vi "PathPlanningSim.vi"() -> ()   [LabVIEW 2019]
uses:
  <vilib>/Analysis/6fits.llb/nD B-Spline Fit.vi
  <vilib>/robotics/Navigation/shared/WorldMap/OccupancyGridWorldMap/NI_Robotics_OccupancyGridWorldMap.lvclass
  <vilib>/Analysis/NI_AALPro.lvlib
panel:
  out "Array":dbl[](array[numeric])
  out "A* Planned\nPath Coordinates":dbl[][](array[numeric])
  in  "stop":bool
  out "Real Occupancy Grid":dbl[][](array[numeric])
  out "Trajectory Plot":cluster{dbl[], dbl[]}[](graph)
  out "Intensity Graph 2":dbl[][](graph) caption="Intensity Graph"
  # "x coordinates"
  # "y coordinates"
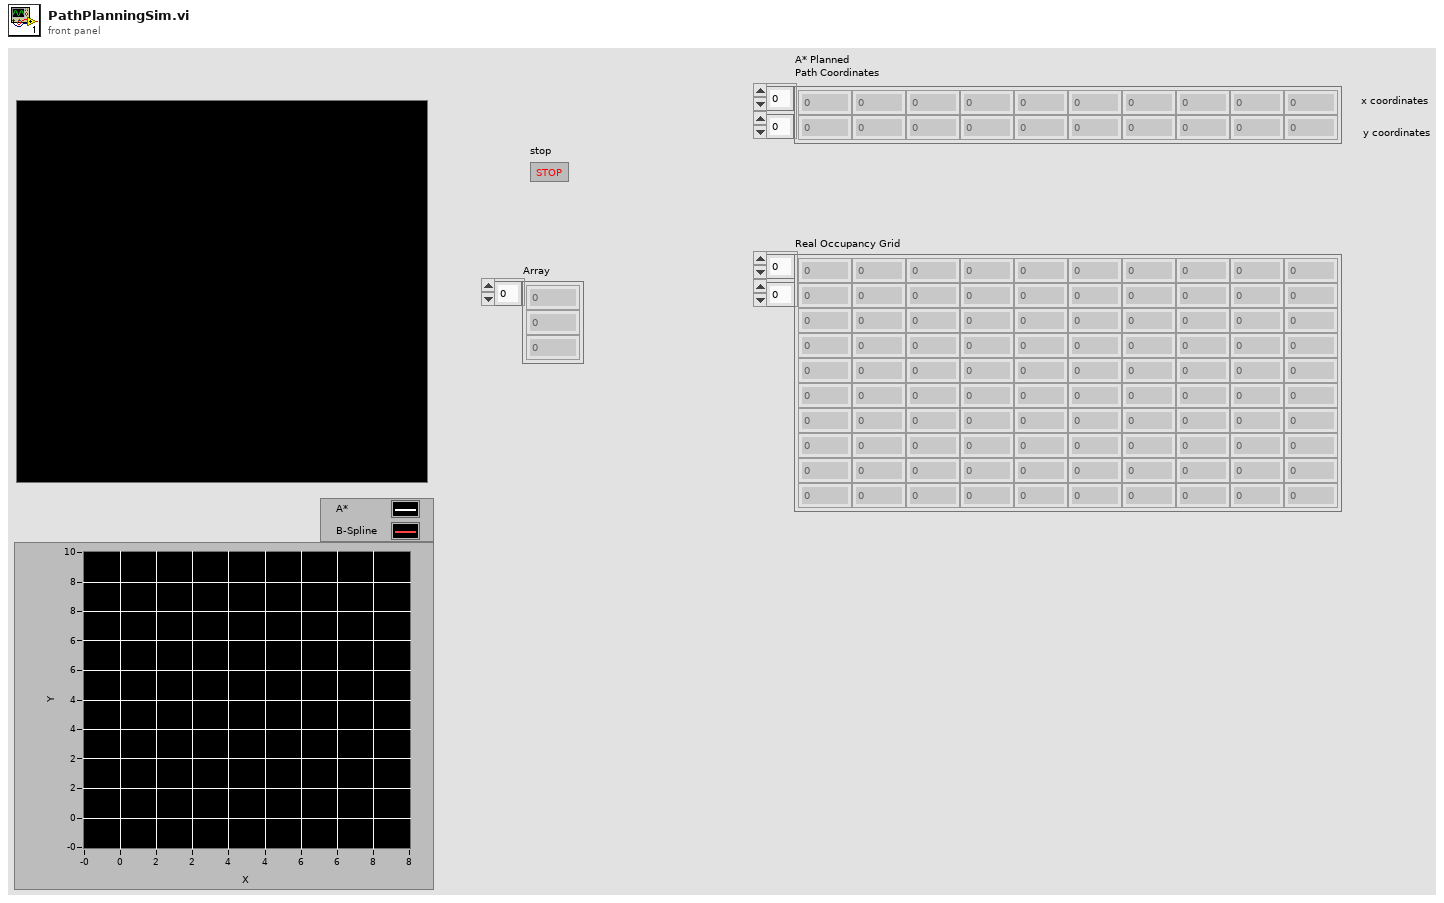
[diagram p1: front panel]
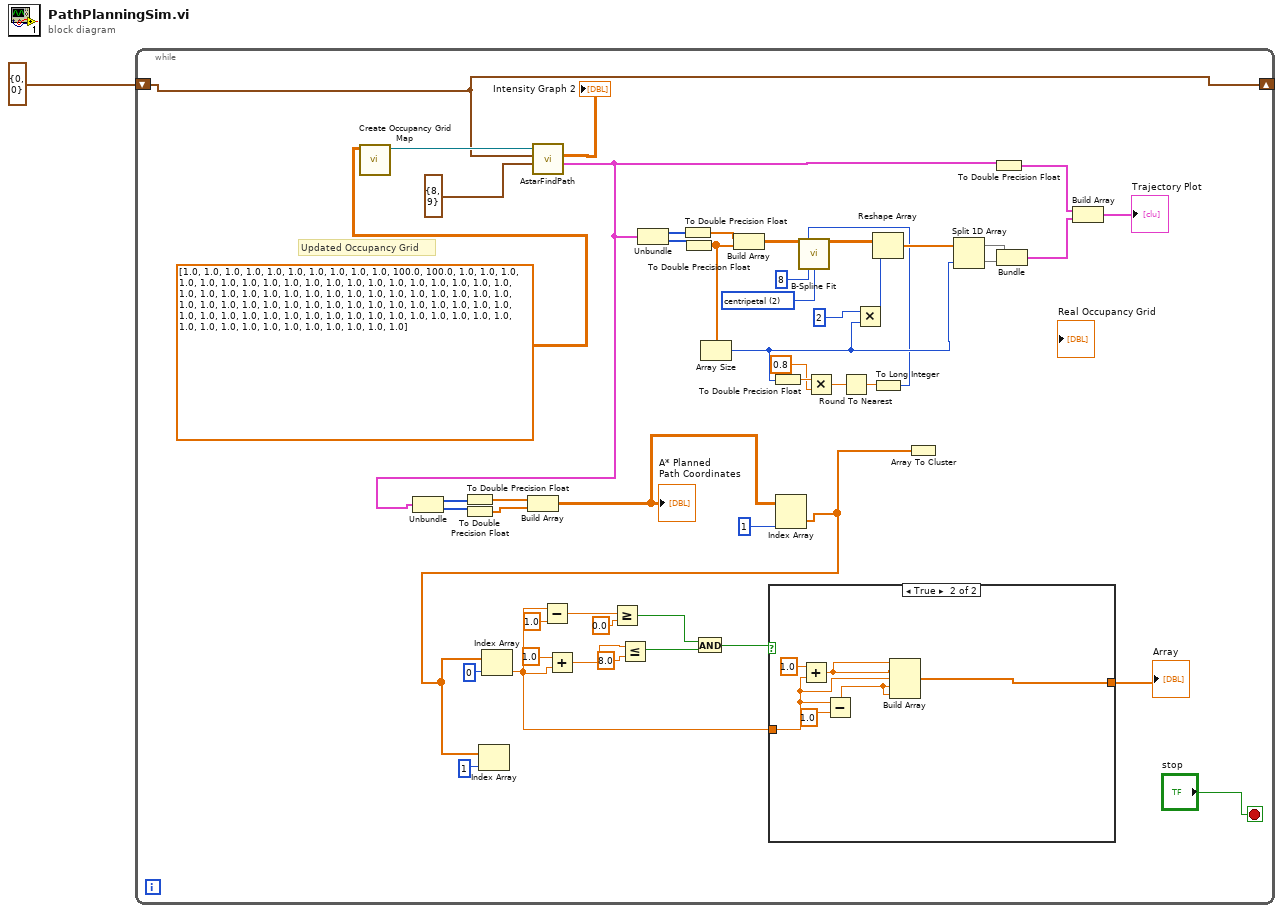
[diagram p0: block diagram]
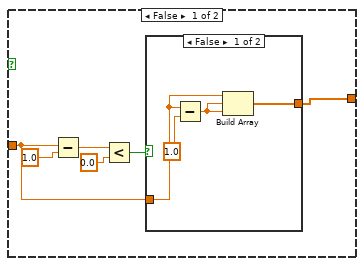
[diagram p2: hidden frame]
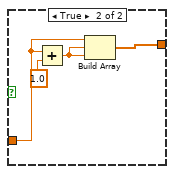
[diagram p3: hidden frame]
diagram:
  n1 = while {
    shift-right: [w4] -> _
    shift-left: cluster{"X":i32, "Y":i32} {"X"=0, "Y"=0} ("goal node") -> [w4]
    stop <- "stop" stop-if-true
    w42 = u16 2 items=["equally spaced", "chord length", "centripetal"] ("parameter selection")
    # "Updated Occupancy Grid"
    n2 = call <vilib>:"Create Occupancy Grid Map.vi"("occupancy grid"=dbl[][] [[1.0, 1.0, 1.0, 1.0, 1.0, 1.0, 1.0, 1.0, 1.0, 1.0], [100.0, 100.0, 1.0, 1.0, 1.0, 1.0, 1.0, 1.0, 1.0, 1.0], [1.0, 1.0, 1.0, 1.0, 1.0, 1.0, 1.0, 1.0, 1.0, 1.0], [1.0, 1.0, 1.0, 1.0, 1.0, 1.0, 1.0, 1.0, 1.0, 1.0], [1.0, 1.0, 1.0, 1.0, 1.0, 1.0, 1.0, 1.0, 1.0, 1.0], [1.0, 1.0, 1.0, 1.0, 1.0, 1.0, 1.0, 1.0, 1.0, 1.0], [1.0, 1.0, 1.0, 1.0, 1.0, 1.0, 1.0, 1.0, 1.0, 1.0], [1.0, 1.0, 1.0, 1.0, 1.0, 1.0, 1.0, 1.0, 1.0, 1.0], [1.0, 1.0, 1.0, 1.0, 1.0, 1.0, 1.0, 1.0, 1.0, 1.0]]) -> ("map reference out"=w50:refnum<data-value>)  [unwired: 9 in, 1 out]
    n3 = call "AstarFindPath.vi"("goal node"=cluster{"X":i32, "Y":i32} {"X"=8, "Y"=9}, "start node"=w4, "map reference in"=w50) -> ("Planned Path"=w19:cluster{i32[], i32[]}, "intensity values"=→"Intensity Graph 2":dbl[][])  [unwired: 5 in, 2 out]
    n4 = Unbundle(w19) -> (w23:i32[], w22:i32[])
    n5 = To Double Precision Float(number=w23) -> (double precision float=w21:dbl[])
    n6 = To Double Precision Float(number=w22) -> (double precision float=w20:dbl[])
    n7 = Build Array(w21, w20) -> (w18:dbl[][])
    "A* Planned\nPath Coordinates" <- w18
    n8 = Unbundle(w19) -> (w47:i32[], w46:i32[])
    n9 = To Double Precision Float(number=w47) -> (double precision float=w45:dbl[])
    n10 = To Double Precision Float(number=w46) -> (double precision float=w37:dbl[])
    n11 = Array Size(array=w37) -> (size(s)=w34:i32)
    n12 = Build Array(w45, w37) -> (w44:dbl[][])
    n13 = To Double Precision Float(number=w34) -> (double precision float=w31:dbl)
    n14 = Index Array(array=w18, index (col)=1 ("x+y")) -> (element=w16:dbl[])  [unwired: 1 in]
    n15 = Index Array(array=w16, index=1 ("x+y")) -> ()  [unwired: 1 out]
    n16 = Index Array(array=w16, index=0 ("x+y")) -> (element=w3:dbl)
    n17 = Subtract(x=w3, y=1.0) -> (x-y=w10:dbl)
    n18 = Add(x=1.0 ("y"), y=w3) -> (x+y=w7:dbl)
    n19 = Greater Or Equal?(x=w10, y=0.0) -> (x >= y?=w5:bool)
    n20 = Less Or Equal?(x=w7, y=8.0) -> (x <= y?=w13:bool)
    n21 = And(x=w5, y=w13) -> (x .and. y?=w12:bool)
    n22 = case shown="True" w12 {
      tunnel: w3 -> [w52 w65]
      tunnel: [w51 w68] -> w2
      frame False {
        n23 = Subtract(x=w52, y=1.0) -> (x-y=w55:dbl)
        n24 = Less?(x=w55, y=0.0) -> (x < y?=w53:bool)
        n25 = case shown="False" w53 {
          tunnel: w52 -> [w58 w63]
          tunnel: [w57 w61] -> w51
          frame False {
            n26 = Subtract(x=w58, y=1.0) -> (x-y=w60:dbl)
            n27 = Build Array(w58, w60, w60) -> (w57:dbl[])
          }
          frame True {
            n28 = Add(x=w63, y=1.0) -> (x+y=w62:dbl)
            n29 = Build Array(w63, w62, w62) -> (w61:dbl[])
          }
        }
      }
      frame True {
        n30 = Add(x=1.0 ("y"), y=w65) -> (x+y=w67:dbl)
        n31 = Subtract(x=w65, y=1.0) -> (x-y=w66:dbl)
        n32 = Build Array(w67, w67, w65, w66, w66) -> (w68:dbl[])
      }
    }
    "Array" <- w2
    n33 = Multiply(x=w31, y=0.8) -> (x*y=w29:dbl)
    n34 = Round To Nearest(number=w29) -> (nearest integer value=w33:dbl)
    n35 = Multiply(x=2, y=w34) -> (x*y=w36:i32)
    n36 = To Long Integer(number=w33) -> (32bit integer=w32:i32)
    n37 = call-poly <vilib>:"B-Spline Fit.vi"("Data"=w44, "# of control points"=w32, "degree"=8, "parameter selection"=w42) -> ("Best BSpline Fit"=w41:dbl[][])  [unwired: 9 in, 2 out]
    n38 = Reshape Array(w41, w36) -> (w40:dbl[])
    n39 = Array To Cluster(array=w16) -> ()  [unwired: 1 out]
    n40 = Split 1D Array(array=w40, index=w34) -> (first subarray=w39:dbl[], second subarray=w38:dbl[])
    n41 = To Double Precision Float(number=w19) -> (double precision float=w27:cluster{dbl[], dbl[]})
    n42 = Bundle(w39, w38) -> (w26:cluster{dbl[], dbl[]})  [unwired: 1 in]
    n43 = Build Array(w27, w26) -> (→"Trajectory Plot":cluster{dbl[], dbl[]}[])
  }
